vi "Init IPC.vi"(8 "error in (no error)":errorcluster, 11 "TCPMessaging in":refnum<class "TCPMessaging.lvclass">) -> (0 "error out":errorcluster, 3 "TCPMessaging out":refnum<class "TCPMessaging.lvclass">)   [LabVIEW 2020, in "Vecto.lvlib" / "TCPMessaging.lvclass"]
uses:
  TCPMessaging.lvclass
  Send Message Data.ctl
  proto/TcpPayload/Data.ctl
  lv-promises/Promises/Promise/Promise.lvclass
  TCPConnectionHandler/TCPConnectionHandler.lvclass
  TCPMessageHandler/TCPMessageHandler.lvclass
  Request Registration.ctl
  Target Group Maps.ctl
  proto/TcpClientList/Data.ctl
  proto/TcpClientInfo/Data.ctl
  TCPMessaging.lvclass/TCPMessaging.ctl
  TX Payload.ctl
  Client Action Data.ctl
  Client Action.ctl
  Client Info.ctl
  VectoConfig/VectoConfig.lvlib
  Vecto.lvlib
  proto/TcpPayload/TcpPayload.lvlib
  TCPMessageService/TCPMessageAPI.lvclass
  proto/TcpClientInfo/TcpClientInfo.lvlib
  proto/TcpClientList/TcpClientList.lvlib
  Connected Status.ctl
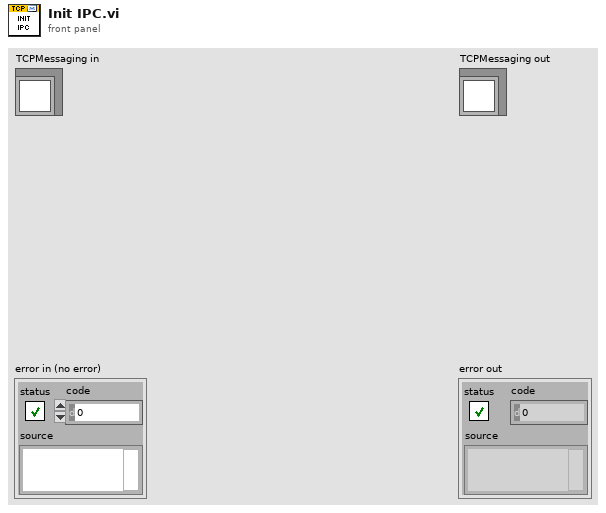
[diagram p1: front panel]
types:
  T1 = typedef "TcpClientList.lvlib/Data.ctl" = cluster{"clients":T2[]}
  T2 = typedef "TcpClientInfo.lvlib/Data.ctl" = cluster{"node_id":u32, "node_name":string, "app_version":string, "config_version":string, "config_hash":string, "node_alias":string, "address":string}
  T3 = typedef "Vecto.lvlib/TCPMessaging.lvclass/Target Group Maps.ctl" = cluster{"Target":map{u32, u32[]}, "Node":map{u32, u32[]}}
  T4 = typedef "Vecto.lvlib/TCPMessaging.lvclass/Request Registration.ctl" = cluster{"Sequence":u32, "Reply Promise":refnum<class "Promise.lvclass">, "Reply Deadline":dbl}
  T5 = typedef "TcpPayload.lvlib/Data.ctl" = cluster{"target_node":u32, "source_id":u32, "sequence":u32, "timestamp":i64, "type":string, "task_id":string, "payload":u8[]}
  T6 = typedef "Vecto.lvlib/Send Message Data.ctl" = cluster{"TcpPayload":T5, "Register Reply":bool, "Reply Promise":refnum<class "Promise.lvclass">, "Reply Deadline":dbl}
  T7 = typedef "Vecto.lvlib/TCPMessaging.lvclass/TCP Mode.ctl" = enum16{"Client", "Server"}
  T8 = typedef "Vecto.lvlib/Connected Status.ctl" = enum16{"Disconnected", "Connected", "Bad Config", "Not Allowed", "Server"}
  T9 = typedef "VectoConfig.lvlib/Client Info.ctl" = cluster{"TcpClientHello":cluster{"node_id":u32, "system":string, "cluster":string, "node_name":string, "app_version":string, "config_version":string, "config_hash":string, "node_alias":string}, "Remote Address":string, "Remote Port":u16}
  T10 = typedef "Vecto.lvlib/TCPMessaging.lvclass/Client Action Data.ctl" = cluster{"Client Action":T11, "Client Info":T9, "TCP":refnum<k5>, "TX Q":refnum<queue>}
  T11 = typedef "Vecto.lvlib/TCPMessaging.lvclass/Client Action.ctl" = enum16{"Connect", "Ready", "Disconnect"}
  T12 = typedef "Vecto.lvlib/TX Payload.ctl" = cluster{"Target ID":u32, "Payload":string}
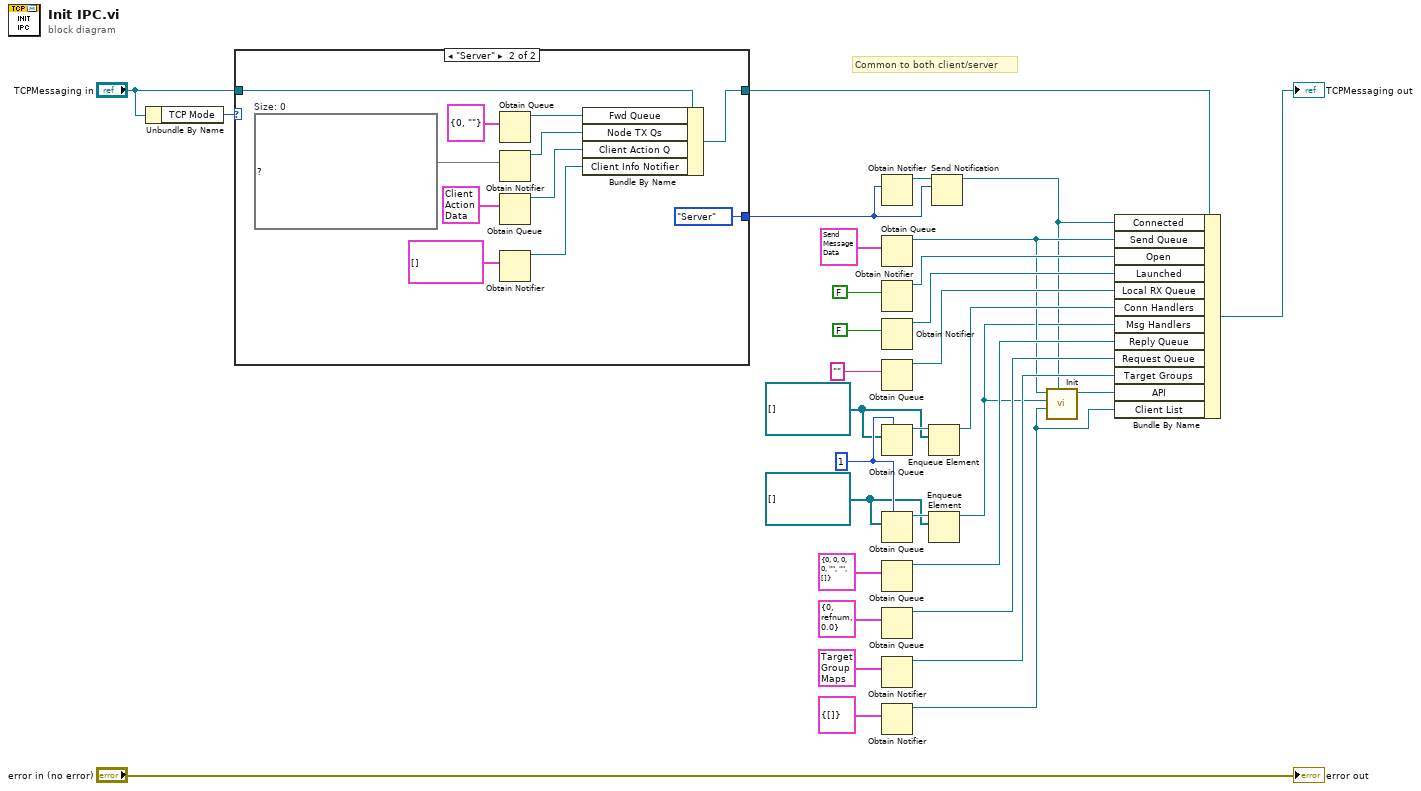
[diagram p0: block diagram]
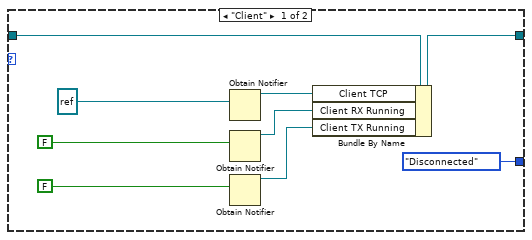
[diagram p2: hidden frame]
diagram:
  w19 = 1 ("max queue size (-1, unlimited)")
  w16 = refnum<class "TCPMessageHandler.lvclass">[] []
  w18 = refnum<class "TCPConnectionHandler.lvclass">[] [] ("Array")
  # "Common to both client/server"
  n1 = Unbundle By Name("TCPMessaging in") -> ("TCP Mode"=w30:T7)
  n2 = case shown="\"Server\"" w30 {
    tunnel: "TCPMessaging in" -> [w40 w52]
    tunnel: [w41 w50] -> w24
    tunnel: [Connected_Status."Disconnected" ("Connected Status") Connected_Status."Server" ("Connected Status")] -> w1
    frame "Client" {
      n3 = Obtain Notifier(notification data type=refnum<k5> refnum ("connection ID")) -> (notifier out=w38:refnum<notifier>)  [unwired: 3 in, 2 out]
      n4 = Obtain Notifier(notification data type=FALSE) -> (notifier out=w36:refnum<notifier>)  [unwired: 3 in, 2 out]
      n5 = Obtain Notifier(notification data type=FALSE) -> (notifier out=w34:refnum<notifier>)  [unwired: 3 in, 2 out]
      n6 = Bundle By Name(cluster=w40, "Client TCP"=w38, "Client RX Running"=w36, "Client TX Running"=w34) -> (w41:refnum<class "TCPMessaging.lvclass">)
    }
    frame "Server" {
      w46 = map{u32, refnum<queue>[]} {}  # Size: 0
      n7 = Obtain Queue(element data type=T12 {"Target ID"=0, "Payload"=""} ("TX Payload")) -> (queue out=w49:refnum<queue>)  [unwired: 4 in, 2 out]
      n8 = Obtain Notifier(notification data type=w46) -> (notifier out=w45:refnum<notifier>)  [unwired: 3 in, 2 out]
      n9 = Obtain Queue(element data type=T10 {"Client Action"=enum."Disconnect", "Client Info"={"TcpClientHello"={"node_id"=0, "system"="", "cluster"="", "node_name"="", "app_version"="", "config_version"="", "config_hash"="", "node_alias"=""}, "Remote Address"="", "Remote Port"=0}, "TCP"=refnum, "TX Q"=refnum} ("Client Action Data")) -> (queue out=w47:refnum<queue>)  [unwired: 4 in, 2 out]
      n10 = Obtain Notifier(notification data type=T9[] []) -> (notifier out=w43:refnum<notifier>)  [unwired: 3 in, 2 out]
      n11 = Bundle By Name(cluster=w52, "Fwd Queue"=w49, "Node TX Qs"=w45, "Client Action Q"=w47, "Client Info Notifier"=w43) -> (w50:refnum<class "TCPMessaging.lvclass">)
    }
  }
  n12 = Obtain Notifier(notification data type=w1) -> (notifier out=w3:refnum<notifier>)  [unwired: 3 in, 2 out]
  n13 = Obtain Queue(element data type=T6 {"TcpPayload"={"target_node"=0, "source_id"=0, "sequence"=0, "timestamp"=0, "type"="", "task_id"="", "payload"=[]}, "Register Reply"=FALSE, "Reply Promise"=refnum, "Reply Deadline"=0.0} ("Send Message Data")) -> (queue out=w8:refnum<queue>)  [unwired: 4 in, 2 out]
  n14 = Obtain Notifier(notification data type=FALSE) -> (notifier out=w29:refnum<notifier>)  [unwired: 3 in, 2 out]
  n15 = Obtain Notifier(notification data type=FALSE) -> (notifier out=w25:refnum<notifier>)  [unwired: 3 in, 2 out]
  n16 = Obtain Queue(element data type="") -> (queue out=w21:refnum<queue>)  [unwired: 4 in, 2 out]
  n17 = Obtain Queue(max queue size (-1, unlimited)=w19, element data type=w18) -> (queue out=w20:refnum<queue>)  [unwired: 3 in, 2 out]
  n18 = Obtain Queue(max queue size (-1, unlimited)=w19, element data type=w16) -> (queue out=w17:refnum<queue>)  [unwired: 3 in, 2 out]
  n19 = Obtain Queue(element data type=T5 {"target_node"=0, "source_id"=0, "sequence"=0, "timestamp"=0, "type"="", "task_id"="", "payload"=[]} ("TcpPayload")) -> (queue out=w13:refnum<queue>)  [unwired: 4 in, 2 out]
  n20 = Obtain Queue(element data type=T4 {"Sequence"=0, "Reply Promise"=refnum, "Reply Deadline"=0.0} ("Request Registration")) -> (queue out=w11:refnum<queue>)  [unwired: 4 in, 2 out]
  n21 = Obtain Notifier(notification data type=T3 {"Target"={}, "Node"={}} ("Target Group Maps")) -> (notifier out=w10:refnum<notifier>)  [unwired: 3 in, 2 out]
  n22 = Obtain Notifier(notification data type=T1 {"clients"=[]} ("TcpClientList")) -> (notifier out=w4:refnum<notifier>)  [unwired: 3 in, 2 out]
  n23 = Enqueue Element(queue=w20, element=w18) -> (queue out=w15:refnum<queue>)  [unwired: 2 in, 2 out]
  n24 = Enqueue Element(queue=w17, element=w16) -> (queue out=w6:refnum<queue>)  [unwired: 2 in, 2 out]
  n25 = Send Notification(notification=w1, notifier=w3) -> (notifier out=w2:refnum<notifier>)  [unwired: 1 in, 1 out]
  n26 = call "Init.vi"("Connection State"=w2, "Client List"=w4, "Msg Handlers"=w6, "Send Queue"=w8) -> ("TCPMessageService out"=w7:refnum<class "TCPMessageAPI.lvclass">)  [unwired: 6 in, 1 out]
  n27 = Bundle By Name(cluster=w24, "Connected"=w2, "Send Queue"=w8, "Open"=w29, "Launched"=w25, "Local RX Queue"=w21, "Conn Handlers"=w15, "Msg Handlers"=w6, "Reply Queue"=w13, "Request Queue"=w11, "Target Groups"=w10, "API"=w7, "Client List"=w4) -> (→"TCPMessaging out":refnum<class "TCPMessaging.lvclass">)
  "error out" <- "error in (no error)"
